vi "Image Display Change Palette.vi"(8 "Error In":errorcluster, 9 "Palette Color":u32, 10 "Color Palette":T2, 11 "Image Control Refnum":T1) -> (0 "Error Out":errorcluster)   [LabVIEW 2021, in "Image.lvlib"]
uses:
  Image.lvlib
  Arrays/Color Palette.ctl
  Image Control Refnum.ctl
  Palette/Palette.lvlib
  <vilib>/vision/NI_Vision_Development_Module.lvlib
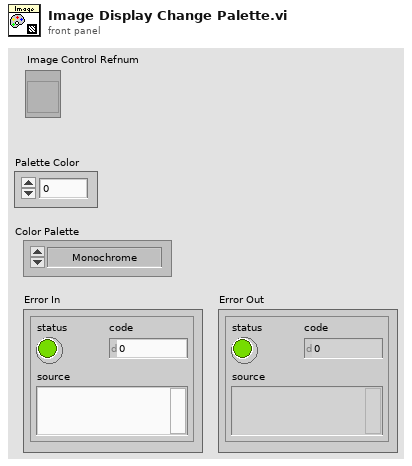
[diagram p1: front panel]
types:
  T1 = typedef "Image.lvlib/Image Control Refnum.ctl" = refnum<vi>
  T2 = typedef "Palette.lvlib/Color Palette.ctl" = enum32{"Monochrome", "Binary", "Gradient", "Rainbow", "Temperature"}
  T3 = cluster{"Red (or Hue) value":u8, "Green (or Sat) value":u8, "Blue (or Light or Val) value":u8}[]
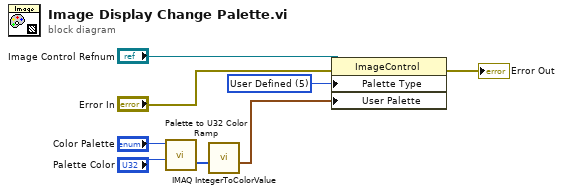
[diagram p0: block diagram]
diagram:
  w7 = u32 5 items=["Grayscale", "Binary", "Gradient", "Rainbow", "Temperature", "User Defined", "Binary 16 Bit", "Gradient 16 Bit", "Rainbow 16 Bit", "Temperature 16 Bit", "User Defined 16 Bit"] ("Palette:Palette Type")
  n1 = call "Palette to U32 Color Ramp.vi"("Color Box"="Palette Color", "Palette"="Color Palette") -> ("Palette Ramp"=w4:u32[])  [unwired: 9 in]
  n2 = call "IMAQ IntegerToColorValue"("1D U32 array"=w4) -> ("1D Color value array"=w3:T3)  [unwired: 4 in, 3 out]
  n3 = property class="ImageControl"(reference="Image Control Refnum", error in="Error In", "Palette Type"=w7, "User Palette"=w3) -> (error out=→"Error Out":errorcluster)  [unwired: 1 out]
